vi "Initialise.vi"(8 "error in (no error)":errorcluster, 11 "LoggingHandle in":refnum<class "LoggingHandle.lvclass">) -> (0 "error out":errorcluster, 3 "LoggingHandle out":refnum<class "LoggingHandle.lvclass">)   [LabVIEW 2024, in "LoggingHandle.lvclass"]
uses:
  LoggingHandle.lvclass
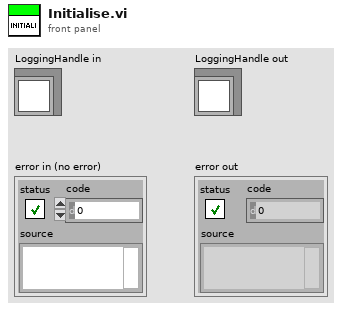
[diagram p1: front panel]
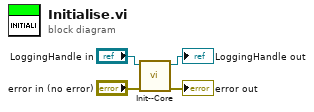
[diagram p0: block diagram]
diagram:
  n1 = call-dynamic "Init--Core.vi"("error in (no error)"="error in (no error)", "LoggingHandle in"="LoggingHandle in") -> ("error out"=→"error out":errorcluster, "LoggingHandle out"=→"LoggingHandle out":refnum<class "LoggingHandle.lvclass">)  [unwired: 8 in]
